vi "Live read with led for drums.vi"() -> ()   [LabVIEW 2009]
uses:
  <vilib>/vision/Image Controls.llb/IMAQ Image.ctl
  <vilib>/Instr/_visa.llb/VISA Configure Serial Port (Instr).vi
  <vilib>/userDefined/High Color/IMAQdx.ctl
  <vilib>/Analysis/3filter.llb/Filter Passband Type.ctl
  <vilib>/Analysis/3filter.llb/Butterworth Filter (DBL).vi
  <vilib>/vision/NI_Vision_Development_Module.lvlib
  <vilib>/Analysis/NI_AALBase.lvlib
  <vilib>/vision/driver/NI_Vision_Acquisition_Software.lvlib
panel:
  in  "Mask":T1 {"Contours"."Type" items=["No Selection", "Point", "Line", "Rectangle", "Oval", "Polygon", "Freehand Region", "Annulus", "Unused2", "Unused3", "Broken Line", "Freehand Line", "Rotated Rectangle"]}
  out "Image 2":T2(plugin-control)
  out "Red Line":T1={"Global Rectangle"=[300, 297, 320, 380], "Contours"=[{"ID"=enum."External", "Type"=2, "Coordinates"=[300, 379, 319, 297]}]} {"Contours"."Type" items=["No Selection", "Point", "Line", "Rectangle", "Oval", "Polygon", "Freehand Region", "Annulus", "Unused2", "Unused3", "Broken Line", "Freehand Line", "Rotated Rectangle"]}
  in  "Red Line":T1={"Global Rectangle"=[300, 297, 320, 380], "Contours"=[{"ID"=enum."External", "Type"=2, "Coordinates"=[300, 379, 319, 297]}]} {"Contours"."Type" items=["No Selection", "Point", "Line", "Rectangle", "Oval", "Polygon", "Freehand Region", "Annulus", "Unused2", "Unused3", "Broken Line", "Freehand Line", "Rotated Rectangle"]}
  out "Waveform Red":dbl[](graph)
  out "LED Red":bool
  in  "sampling 4":dbl=1.0 format="%0.2f"
  in  "high 4":dbl=60.0 format="%0.2f"
  in  "low  4":dbl=0.12500000000000006 format="%0.4f"
  out "Green Line":T1={"Global Rectangle"=[406, 309, 423, 383], "Contours"=[{"ID"=enum."External", "Type"=2, "Coordinates"=[422, 382, 406, 309]}]} {"Contours"."Type" items=["No Selection", "Point", "Line", "Rectangle", "Oval", "Polygon", "Freehand Region", "Annulus", "Unused2", "Unused3", "Broken Line", "Freehand Line", "Rotated Rectangle"]}
  in  "Blue Line":T1={"Global Rectangle"=[374, 278, 383, 377], "Contours"=[{"ID"=enum."External", "Type"=2, "Coordinates"=[382, 376, 374, 278]}]} {"Contours"."Type" items=["No Selection", "Point", "Line", "Rectangle", "Oval", "Polygon", "Freehand Region", "Annulus", "Unused2", "Unused3", "Broken Line", "Freehand Line", "Rotated Rectangle"]}
  in  "Green Line":T1={"Global Rectangle"=[406, 309, 423, 383], "Contours"=[{"ID"=enum."External", "Type"=2, "Coordinates"=[422, 382, 406, 309]}]} {"Contours"."Type" items=["No Selection", "Point", "Line", "Rectangle", "Oval", "Polygon", "Freehand Region", "Annulus", "Unused2", "Unused3", "Broken Line", "Freehand Line", "Rotated Rectangle"]}
  in  "low  3":dbl=0.12500000000000006 format="%0.4f"
  out "Waveform Green":dbl[](graph)
  out "LED Green":bool
  in  "sampling 3":dbl=1.0 format="%0.2f"
  in  "high 3":dbl=60.0 format="%0.2f"
  in  "Yellow Line":T1={"Global Rectangle"=[342, 292, 349, 377], "Contours"=[{"ID"=enum."External", "Type"=2, "Coordinates"=[342, 376, 348, 292]}]} {"Contours"."Type" items=["No Selection", "Point", "Line", "Rectangle", "Oval", "Polygon", "Freehand Region", "Annulus", "Unused2", "Unused3", "Broken Line", "Freehand Line", "Rotated Rectangle"]}
  out "Blue Line":T1={"Global Rectangle"=[168, 264, 180, 378], "Contours"=[{"ID"=enum."External", "Type"=2, "Coordinates"=[168, 377, 179, 264]}]} {"Contours"."Type" items=["No Selection", "Point", "Line", "Rectangle", "Oval", "Polygon", "Freehand Region", "Annulus", "Unused2", "Unused3", "Broken Line", "Freehand Line", "Rotated Rectangle"]}
  out "cluster":T3
  in  "baud rate (9600)":u32=9600
  in  "VISA resource name":refnum<visa-resource-name>
  out "number":u32
  out "decimal integer string":string
  out "Image Dst Out":T2
  out "Yellow Line":T1={"Global Rectangle"=[243, 262, 261, 384], "Contours"=[{"ID"=enum."External", "Type"=2, "Coordinates"=[260, 383, 243, 262]}]} {"Contours"."Type" items=["No Selection", "Point", "Line", "Rectangle", "Oval", "Polygon", "Freehand Region", "Annulus", "Unused2", "Unused3", "Broken Line", "Freehand Line", "Rotated Rectangle"]}
  in  "low  2":dbl=0.12500000000000006 format="%0.4f"
  in  "high 2":dbl=60.0 format="%0.2f"
  in  "sampling 2":dbl=1.0 format="%0.2f"
  out "LED Yellow":bool
  out "Waveform Yellow":dbl[](graph)
  in  "playtime":dbl=30.0
  out "Frame Number":i32
  in  "Frame Start":i32=2400
  out "LED BLUE":bool
  in  "low":dbl=0.12500000000000006 format="%0.4f"
  out "Waveform Blue":dbl[](graph)
  in  "high":dbl=60.0 format="%0.2f"
  in  "sampling":dbl=1.0 format="%0.2f"
  in  "stop":bool
  # "BLUE"
  # "YELLOW"
  # "GREEN"
  # "RED"
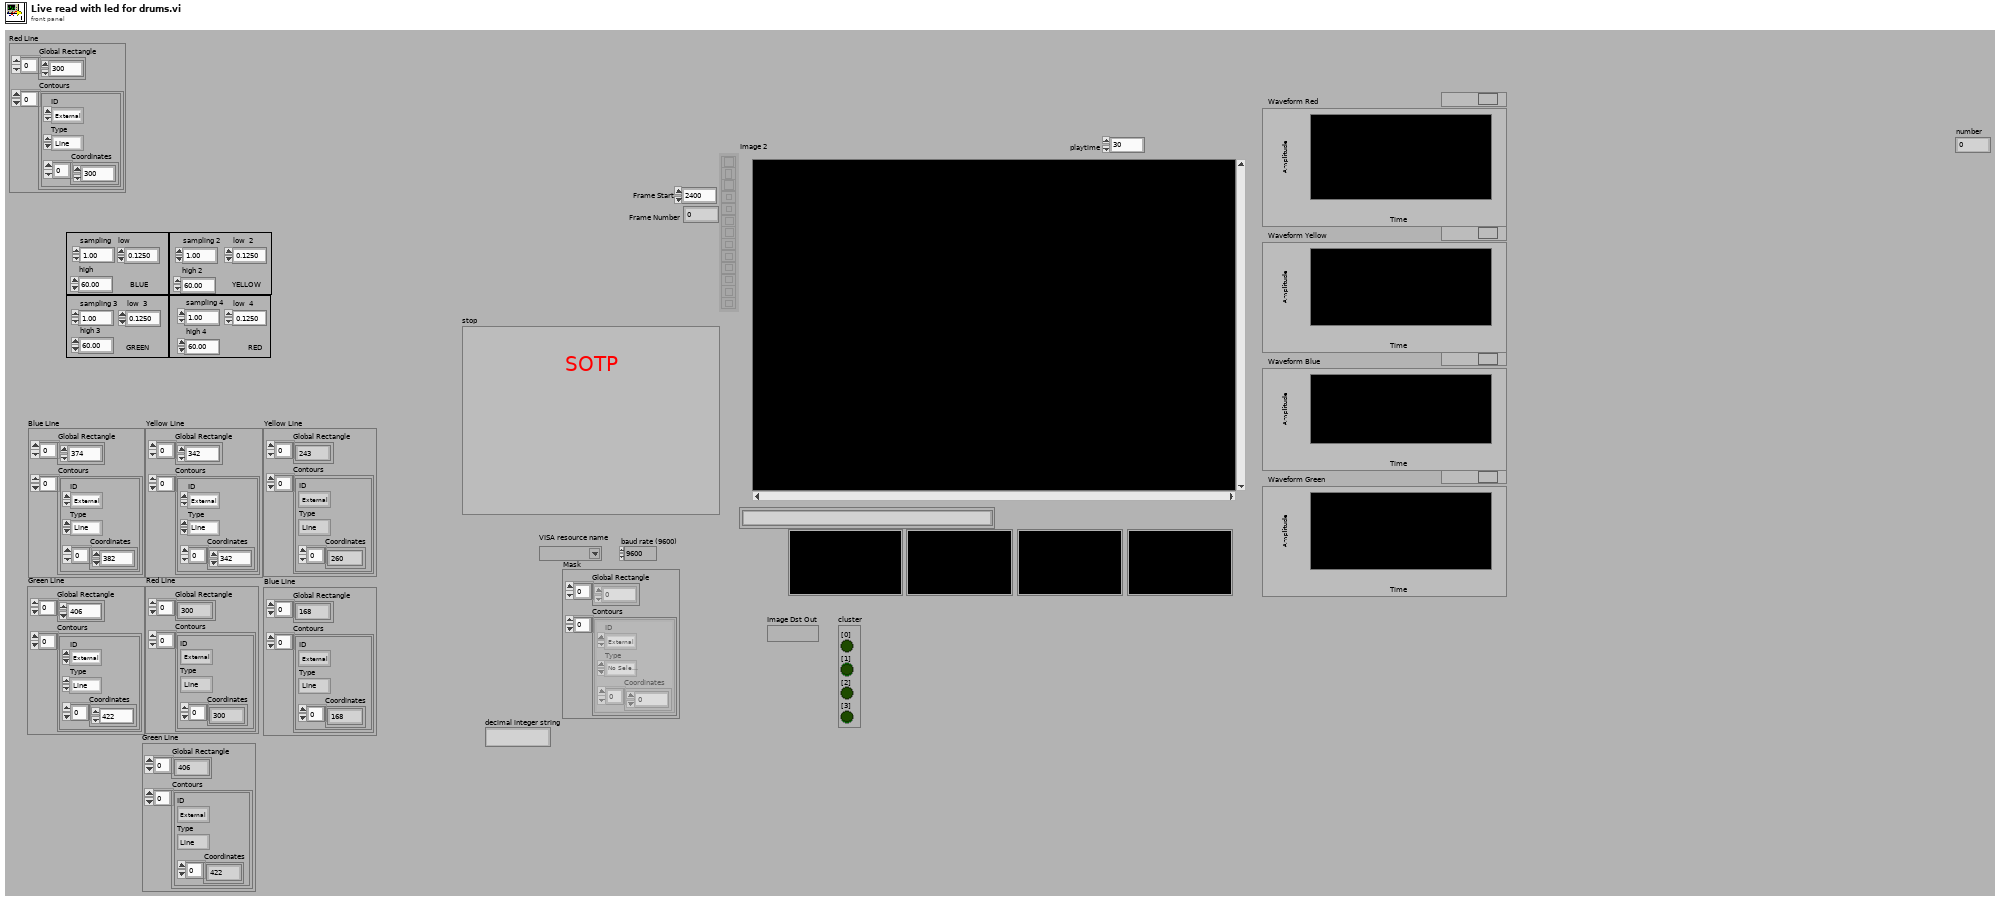
[diagram p1: front panel]
types:
  T1 = cluster{"Global Rectangle":i32[], "Contours":cluster{"ID":enum32{"External", "Internal"}, "Type":u32, "Coordinates":i32[]}[]}
  T2 = typedef "IMAQ Image.ctl" = refnum<image>
  T3 = cluster{"[0]":bool, "[1]":bool, "[2]":bool, "[3]":bool, "[4]":bool, "[5]":bool, "[6]":bool, "[7]":bool, "[8]":bool}
  T4 = typedef "IMAQdx.ctl" = refnum<k21>
  T5 = typedef "NI_AALBase.lvlib/Filter Passband Type.ctl" = enum32{"Lowpass", "Highpass", "Bandpass", "Bandstop"}
  T6 = cluster{"Left":i32, "Top":i32, "Right":i32, "Bottom":i32}
  T7 = typedef "Image Type" = u32
  T8 = cluster{"ID":enum32{"External", "Internal"}, "Type":u32, "Coordinates":i32[]}[]
  T9 = cluster{"ID":enum32{"External", "Internal"}, "Type":u32, "Coordinates":i32[]}
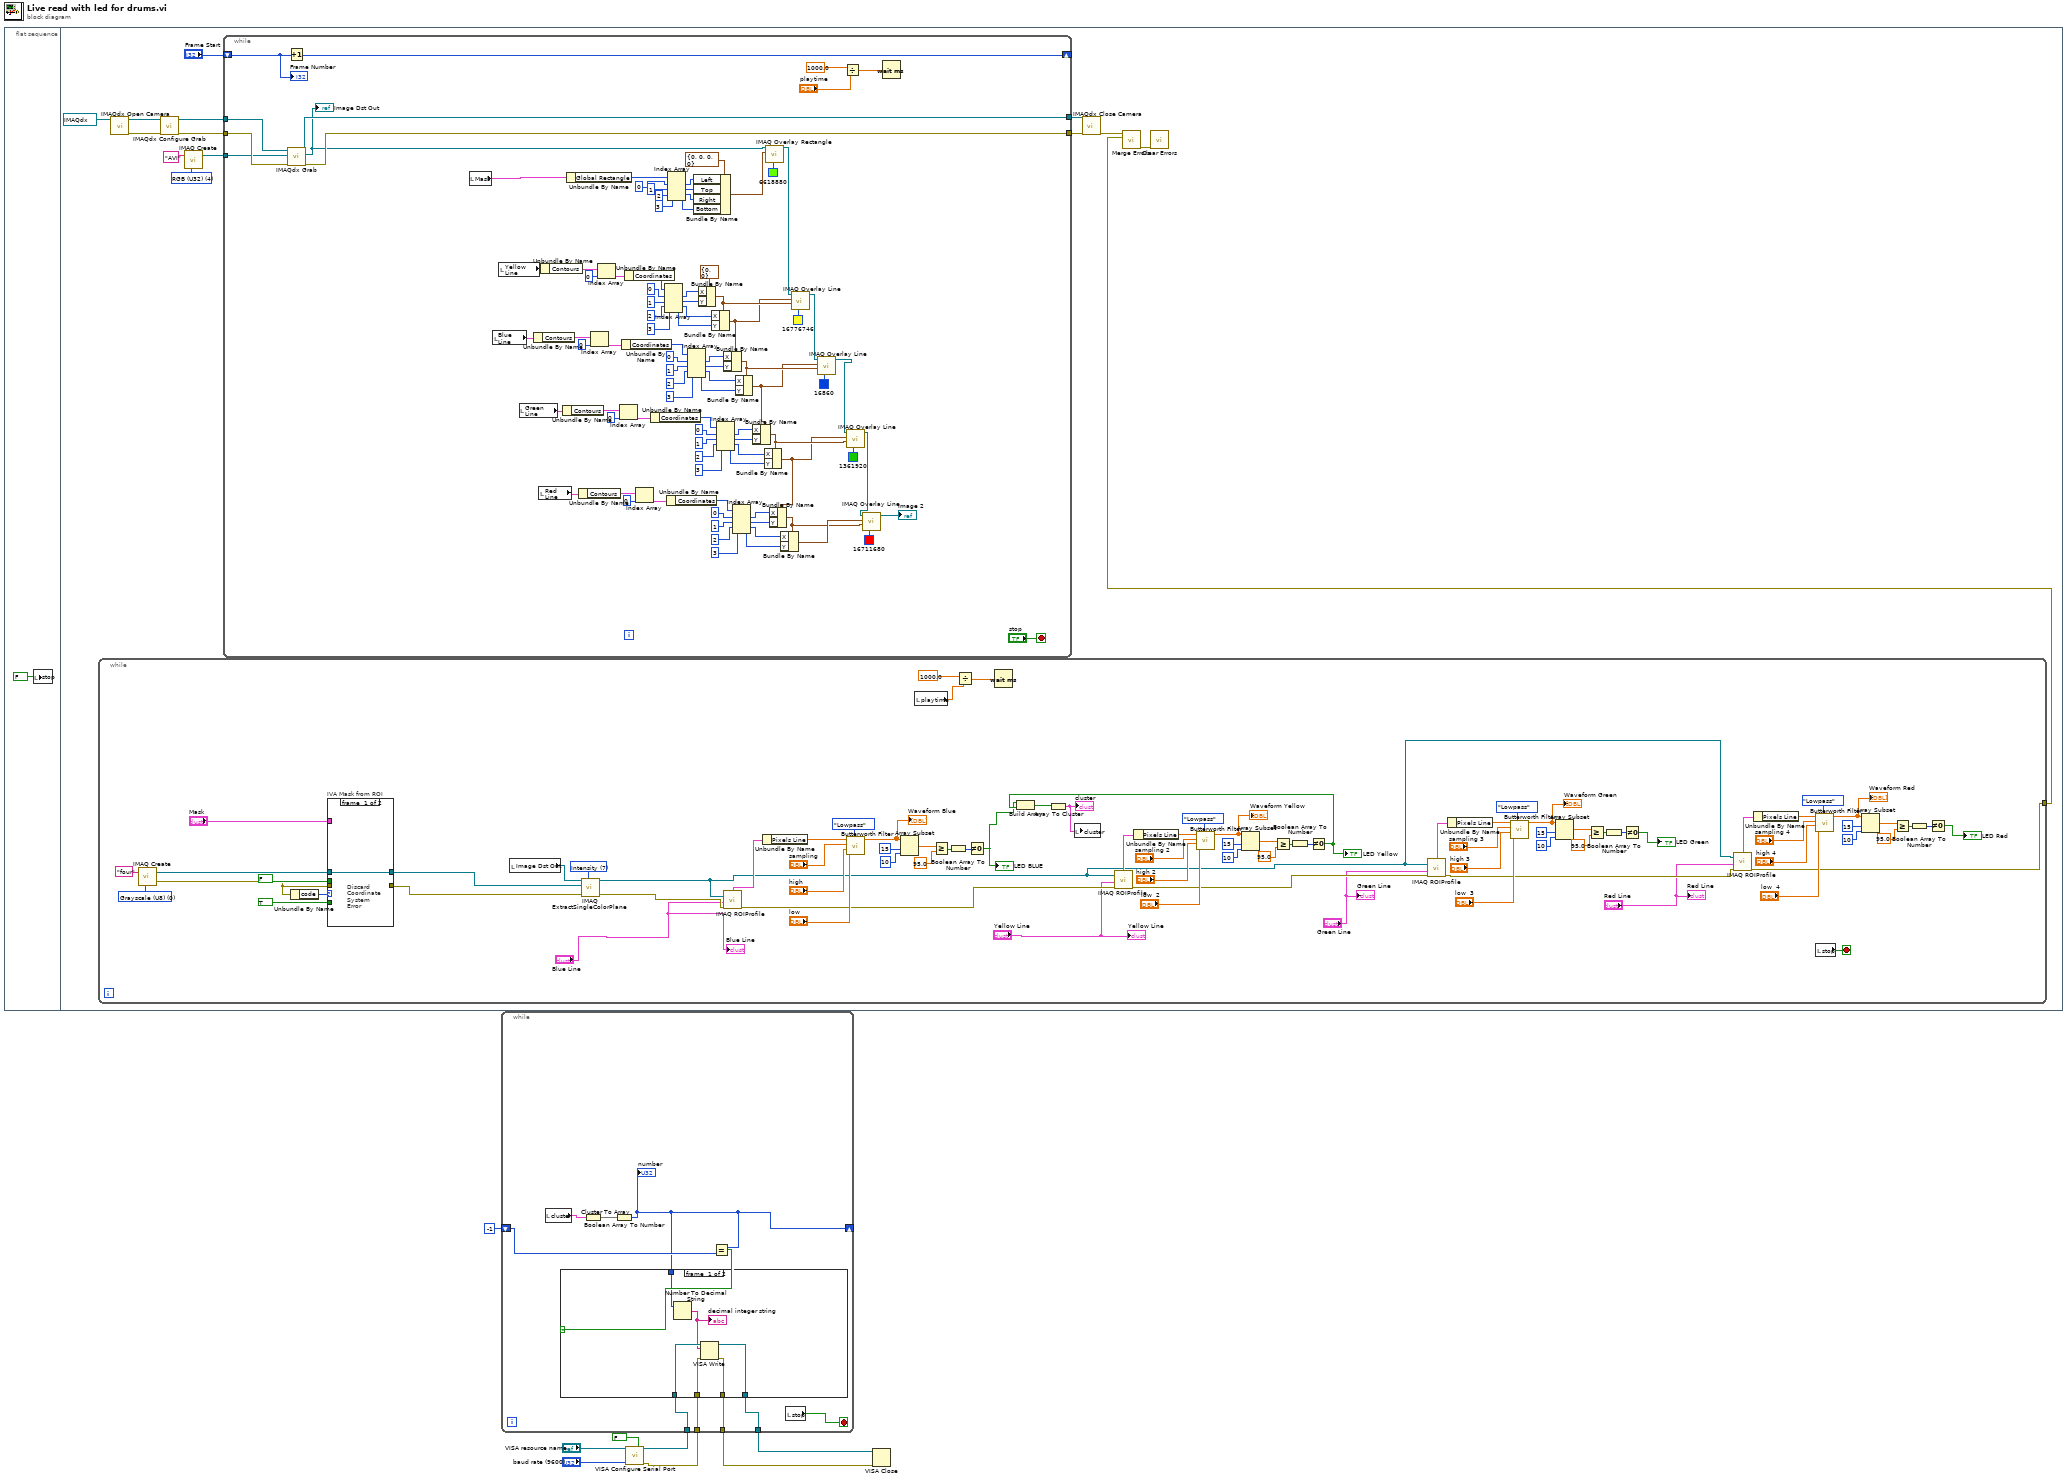
[diagram p0: block diagram]
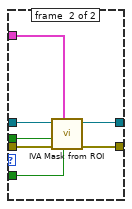
[diagram p3: hidden frame]
diagram:
  n1 = flat-sequence {
    frame #0 {
      n2 = local write "stop"(FALSE ("stop")) -> ()
    }
    frame #1 {
      w21 = T7 4 items=["Grayscale (U8)", "Grayscale (I16)", "Grayscale (SGL)", "Complex (CSG)", "RGB (U32)", "HSL (U32)", "RGB (U64)", "Grayscale (U16)"] ("Image Type")
      n3 = while {
        tunnel: [w34] -> w18
        stop <- w106 stop-if-true
        w77 = T7 0 items=["Grayscale (U8)", "Grayscale (I16)", "Grayscale (SGL)", "Complex (CSG)", "RGB (U32)", "HSL (U32)", "RGB (U64)", "Grayscale (U16)"] ("Image Type")
        w107 = 7 items=["Red", "Green", "Blue", "Hue", "Saturation", "Luminance", "Value", "Intensity"] ("Color Plane")
        n4 = call "IMAQ Create"("Image Name"="four", "Image Type"=w77) -> ("New Image"=w26:T2, "error out"=w27:errorcluster)  [unwired: 3 in]
        n5 = Unbundle By Name(w27) -> ("code"=w31:i32)
        n6 = case "IVA Mask from ROI" shown="Default" w31 {
          tunnel: "Mask" -> [_ w115]
          tunnel: TRUE ("Shrink") -> [_ w114]
          tunnel: w26 -> [w108 w113]
          tunnel: w27 -> [_ w112]
          tunnel: [_ w111] -> w28
          tunnel: [w108 w110] -> w24
          tunnel: FALSE ("Out / In") -> [_ w109]
          frame #0 {
            # "Discard\nCoordinate\nSystem\nError"
          }
          frame #1 {
            n7 = call <vilib>:"IVA Mask from ROI.vi"("Shrink"=w114, "ROI Descriptor"=w115, "error in (no error)"=w112, "Out / In"=w109, "Image Src"=w113) -> ("error out"=w111:errorcluster, "Image Out"=w110:T2)  [unwired: 5 out]
          }
        }
        n8 = local read "Image Dst Out"() -> (w78:T2)
        n9 = call "IMAQ ExtractSingleColorPlane"("Color Plane"=w107, "error in (no error)"=w28, "Image Dst"=w24, "Image Src"=w78) -> ("error out"=w70:errorcluster, "Image Dst Out"=w32:T2)  [unwired: 6 out]
        n10 = call "IMAQ ROIProfile"("error in (no error)"=w70, "ROI Descriptor"="Blue Line", "Image"=w32) -> ("error out"=w71:errorcluster, "ROI Graph"=w69:cluster{"x0":sgl, "dx":sgl, "Pixels Line":sgl[]})  [unwired: 4 out]
        n11 = Unbundle By Name(w69) -> ("Pixels Line"=w104:sgl[])
        n12 = call-poly <vilib>:"Butterworth Filter.vi"("filter type"=Filter_Passband_Type."Lowpass", "low cutoff freq: fl"="low", "high cutoff freq: fh"="high", "sampling freq: fs"="sampling", "X"=w104) -> ("Filtered X"=w51:dbl[])  [unwired: 3 in, 1 out]
        "Waveform Blue" <- w51
        n13 = Array Subset(array=w51, index=15, length=10) -> (w98:dbl[])
        n14 = local read "playtime"() -> (w92:dbl)
        n15 = Greater Or Equal?(x=w98, y=95.0) -> (x >= y?=w96:bool[])
        n16 = Boolean Array To Number(Boolean array=w96) -> (number=w93:u32)
        n17 = Divide(x=1000.0, y=w92) -> (x/y=w95:dbl)
        n18 = Not Equal To 0?(x=w93) -> (x != 0?=w72:bool)
        "LED BLUE" <- w72
        n19 = Wait (ms)(milliseconds to wait=w95) -> ()  [unwired: 1 out]
        n20 = call "IMAQ ROIProfile"("error in (no error)"=w71, "ROI Descriptor"="Yellow Line", "Image"=w32) -> ("error out"=w54:errorcluster, "ROI Graph"=w81:cluster{"x0":sgl, "dx":sgl, "Pixels Line":sgl[]})  [unwired: 4 out]
        n21 = Unbundle By Name(w81) -> ("Pixels Line"=w84:sgl[])
        n22 = call-poly <vilib>:"Butterworth Filter.vi"("filter type"=Filter_Passband_Type."Lowpass", "low cutoff freq: fl"="low  2", "high cutoff freq: fh"="high 2", "sampling freq: fs"="sampling 2", "X"=w84) -> ("Filtered X"=w80:dbl[])  [unwired: 3 in, 1 out]
        "Waveform Yellow" <- w80
        n23 = Array Subset(array=w80, index=15, length=10) -> (w89:dbl[])
        n24 = Greater Or Equal?(x=w89, y=95.0) -> (x >= y?=w87:bool[])
        n25 = Boolean Array To Number(Boolean array=w87) -> (number=w86:u32)
        n26 = Not Equal To 0?(x=w86) -> (x != 0?=w73:bool)
        "LED Yellow" <- w73
        n27 = Build Array(w72, w73) -> (w75:bool[])
        n28 = Array To Cluster(array=w75) -> (cluster=w74:T3)
        "cluster" <- w74
        n29 = local write "cluster"(w74) -> ()
        n30 = call "IMAQ ROIProfile"("error in (no error)"=w54, "ROI Descriptor"="Green Line", "Image"=w32) -> ("error out"=w36:errorcluster, "ROI Graph"=w66:cluster{"x0":sgl, "dx":sgl, "Pixels Line":sgl[]})  [unwired: 4 out]
        n31 = Unbundle By Name(w66) -> ("Pixels Line"=w63:sgl[])
        n32 = call-poly <vilib>:"Butterworth Filter.vi"("filter type"=Filter_Passband_Type."Lowpass", "low cutoff freq: fl"="low  3", "high cutoff freq: fh"="high 3", "sampling freq: fs"="sampling 3", "X"=w63) -> ("Filtered X"=w67:dbl[])  [unwired: 3 in, 1 out]
        "Waveform Green" <- w67
        n33 = Array Subset(array=w67, index=15, length=10) -> (w58:dbl[])
        n34 = Greater Or Equal?(x=w58, y=95.0) -> (x >= y?=w60:bool[])
        n35 = Boolean Array To Number(Boolean array=w60) -> (number=w61:u32)
        n36 = Not Equal To 0?(x=w61) -> (x != 0?=→"LED Green":bool)
        n37 = call "IMAQ ROIProfile"("error in (no error)"=w36, "ROI Descriptor"="Red Line", "Image"=w32) -> ("error out"=w34:errorcluster, "ROI Graph"=w38:cluster{"x0":sgl, "dx":sgl, "Pixels Line":sgl[]})  [unwired: 4 out]
        n38 = Unbundle By Name(w38) -> ("Pixels Line"=w41:sgl[])
        n39 = call-poly <vilib>:"Butterworth Filter.vi"("filter type"=Filter_Passband_Type."Lowpass", "low cutoff freq: fl"="low  4", "high cutoff freq: fh"="high 4", "sampling freq: fs"="sampling 4", "X"=w41) -> ("Filtered X"=w37:dbl[])  [unwired: 3 in, 1 out]
        "Waveform Red" <- w37
        n40 = local read "stop"() -> (w106:bool)
        n41 = Array Subset(array=w37, index=15, length=10) -> (w46:dbl[])
        n42 = Greater Or Equal?(x=w46, y=95.0) -> (x >= y?=w44:bool[])
        n43 = Boolean Array To Number(Boolean array=w44) -> (number=w43:u32)
        n44 = Not Equal To 0?(x=w43) -> (x != 0?=→"LED Red":bool)
        "Yellow Line" <- "Yellow Line"
        "Blue Line" <- "Blue Line"
        "Green Line" <- "Green Line"
        "Red Line" <- "Red Line"
      }
      n45 = call <vilib>:"IMAQdx Open Camera.vi"("Session In"=T4 "cam1") -> ("error out"=w15:errorcluster, "Session Out"=w16:T4)  [unwired: 9 in]
      n46 = call <vilib>:"IMAQdx Configure Grab.vi"("error in"=w15, "Session In"=w16) -> ("error out"=w13:errorcluster, "Session Out"=w14:T4)  [unwired: 8 in]
      n47 = call "IMAQ Create"("Image Name"="AVI", "Image Type"=w21) -> ("New Image"=w19:T2)  [unwired: 3 in, 1 out]
      n48 = while {
        tunnel: w14 -> [w121]
        tunnel: w13 -> [w120]
        shift-right: [w206] -> _
        shift-left: "Frame Start" -> [w205]
        tunnel: [w119] -> w12
        tunnel: w19 -> [w118]
        tunnel: [w117] -> w10
        stop <- "stop" stop-if-true
        n49 = Increment(x=w205) -> (x+1=w206:i32)
        n50 = call <vilib>:"IMAQdx Grab.vi"("error in"=w120, "Image In"=w118, "Session In"=w121) -> ("error out"=w119:errorcluster, "Image Out"=w116:T2, "Session Out"=w117:T4)  [unwired: 5 in, 1 out]
        "Image Dst Out" <- w116
        n51 = local read "Mask"() -> (w122:T1)
        n52 = local read "Blue Line"() -> (w160:T1)
        n53 = local read "Yellow Line"() -> (w159:T1)
        n54 = local read "Green Line"() -> (w158:T1)
        n55 = Unbundle By Name(w160) -> ("Contours"=w172:T8)
        n56 = local read "Red Line"() -> (w125:T1)
        n57 = Unbundle By Name(w159) -> ("Contours"=w187:T8)
        n58 = Unbundle By Name(w158) -> ("Contours"=w148:T8)
        n59 = Unbundle By Name(w122) -> ("Global Rectangle"=w201:i32[])
        n60 = Unbundle By Name(w125) -> ("Contours"=w135:T8)
        n61 = Index Array(array=w172, index=0) -> (element=w171:T9)
        n62 = Index Array(array=w187, index=0) -> (element=w189:T9)
        n63 = Index Array(array=w148, index=0) -> (element=w149:T9)
        n64 = Unbundle By Name(w171) -> ("Coordinates"=w170:i32[])
        n65 = Unbundle By Name(w189) -> ("Coordinates"=w190:i32[])
        n66 = Index Array(array=w135, index=0) -> (element=w134:T9)
        n67 = Unbundle By Name(w149) -> ("Coordinates"=w150:i32[])
        n68 = Index Array(array=w190, index #1=0 ("index"), index #2=1 ("index"), index #3=2 ("index"), index #4=3 ("index")) -> (element #1=w182:i32, element #2=w183:i32, element #3=w184:i32, element #4=w185:i32)
        n69 = Unbundle By Name(w134) -> ("Coordinates"=w133:i32[])
        n70 = Index Array(array=w201, index #1=0 ("index"), index #2=1 ("index"), index #3=2 ("index"), index #4=3 ("index")) -> (element #1=w200:i32, element #2=w199:i32, element #3=w198:i32, element #4=w197:i32)
        n71 = Index Array(array=w170, index #1=0 ("index"), index #2=1 ("index"), index #3=2 ("index"), index #4=3 ("index")) -> (element #1=w169:i32, element #2=w175:i32, element #3=w174:i32, element #4=w173:i32)
        n72 = Bundle By Name(cluster=T6 {"Left"=0, "Top"=0, "Right"=0, "Bottom"=0} ("Rectangle"), "Left"=w200, "Top"=w199, "Right"=w198, "Bottom"=w197) -> (w203:T6)
        n73 = Bundle By Name(cluster=cluster{"X":i32, "Y":i32} {"X"=0, "Y"=0} ("End Point"), "X"=w182, "Y"=w183) -> (w191:cluster{"X":i32, "Y":i32})
        n74 = Bundle By Name(cluster=w191, "X"=w184, "Y"=w185) -> (w162:cluster{"X":i32, "Y":i32})
        n75 = Index Array(array=w150, index #1=0 ("index"), index #2=1 ("index"), index #3=2 ("index"), index #4=3 ("index")) -> (element #1=w151:i32, element #2=w145:i32, element #3=w146:i32, element #4=w147:i32)
        n76 = Bundle By Name(cluster=w162, "X"=w169, "Y"=w175) -> (w176:cluster{"X":i32, "Y":i32})
        n77 = Index Array(array=w133, index #1=0 ("index"), index #2=1 ("index"), index #3=2 ("index"), index #4=3 ("index")) -> (element #1=w132:i32, element #2=w138:i32, element #3=w137:i32, element #4=w136:i32)
        n78 = Bundle By Name(cluster=w176, "X"=w174, "Y"=w173) -> (w143:cluster{"X":i32, "Y":i32})
        n79 = Bundle By Name(cluster=w143, "X"=w151, "Y"=w145) -> (w142:cluster{"X":i32, "Y":i32})
        n80 = Bundle By Name(cluster=w142, "X"=w146, "Y"=w147) -> (w124:cluster{"X":i32, "Y":i32})
        n81 = call "IMAQ Overlay Rectangle"("Color"=u32 6618880, "Rectangle"=w203, "Image"=w116) -> ("Image Out"=w177:T2)  [unwired: 7 in, 1 out]
        n82 = Bundle By Name(cluster=w124, "X"=w132, "Y"=w138) -> (w140:cluster{"X":i32, "Y":i32})
        n83 = Bundle By Name(cluster=w140, "X"=w137, "Y"=w136) -> (w141:cluster{"X":i32, "Y":i32})
        n84 = call "IMAQ Overlay Line"("Color"=u32 16776746, "End Point"=w191, "Start Point"=w162, "Image"=w177) -> ("Image Out"=w167:T2)  [unwired: 6 in, 1 out]
        n85 = call "IMAQ Overlay Line"("Color"=u32 16860, "End Point"=w176, "Start Point"=w143, "Image"=w167) -> ("Image Out"=w144:T2)  [unwired: 6 in, 1 out]
        n86 = Divide(x=1000.0, y="playtime") -> (x/y=w209:dbl)
        n87 = call "IMAQ Overlay Line"("Color"=u32 1361920, "End Point"=w142, "Start Point"=w124, "Image"=w144) -> ("Image Out"=w123:T2)  [unwired: 6 in, 1 out]
        n88 = call "IMAQ Overlay Line"("Color"=u32 16711680, "End Point"=w140, "Start Point"=w141, "Image"=w123) -> ("Image Out"=→"Image 2":T2)  [unwired: 6 in, 1 out]
        n89 = Wait (ms)(milliseconds to wait=w209) -> ()  [unwired: 1 out]
        "Frame Number" <- w205
      }
      n90 = call <vilib>:"IMAQdx Close Camera.vi"("error in"=w12, "Session In"=w10) -> ("error out"=w11:errorcluster)  [unwired: 9 in]
      n91 = call <vilib>:"Merge Errors.vi"("error in 2 (no error)"=w18, "error in 1 (no error)"=w11) -> ("error out"=w22:errorcluster)  [unwired: 5 in]
      n92 = call <vilib>:"Clear Errors.vi"("error in (no error)"=w22) -> ()  [unwired: 6 in, 1 out]
    }
  }
  n93 = call-poly "VISA Configure Serial Port"("VISA resource name"="VISA resource name", "Enable Termination\nChar (T)"=FALSE ("Enable Termination\nChar (T)"), "baud rate (9600)"="baud rate (9600)") -> ("VISA resource name out"=w7:refnum<visa-resource-name>, "error out"=w2:errorcluster)  [unwired: 11 in]
  n94 = while {
    shift-right: [w214] -> _
    shift-left: -1 -> [w220]
    tunnel: w7 -> [w218]
    tunnel: [w217] -> w6
    tunnel: w2 -> [w216]
    tunnel: [w215] -> w1
    stop <- w211 stop-if-true
    n95 = local read "cluster"() -> (w212:T3)
    n96 = Cluster To Array(cluster=w212) -> (array=w213:bool[])
    n97 = Boolean Array To Number(Boolean array=w213) -> (number=w214:u32)
    "number" <- w214
    n98 = Equal?(x=w214, y=w220) -> (x = y?=w219:bool)
    n99 = case shown="False" w219 {
      tunnel: w218 -> [w226 w228]
      tunnel: [w225 w228] -> w217
      tunnel: w214 -> [w223 _]
      tunnel: w216 -> [w222 w227]
      tunnel: [w221 w227] -> w215
      frame #0 {
        n100 = Number To Decimal String(number=w223) -> (decimal integer string=w224:string)  [unwired: 1 in]
        "decimal integer string" <- w224
        n101 = VISA Write(VISA resource name=w226, write buffer=w224, error in (no error)=w222) -> (VISA resource name out=w225:refnum<visa-resource-name>, error out=w221:errorcluster)  [unwired: 1 out]
      }
      frame #1 {
      }
    }
    n102 = local read "stop"() -> (w211:bool)
  }
  n103 = VISA Close(VISA resource name=w6, error in (no error)=w1) -> ()  [unwired: 1 out]
